vi "Thermometer_Property Node Demo.vi"() -> ()   [LabVIEW 2010]
panel:
  in  "Stop Button":bool
  in  "Temperature":dbl format="%.2g"
  out "Thermometer":dbl(slide) scale=0.0..100.0
  # "The color of the thermometer changes\nwhen the temperature is above 50 degrees."
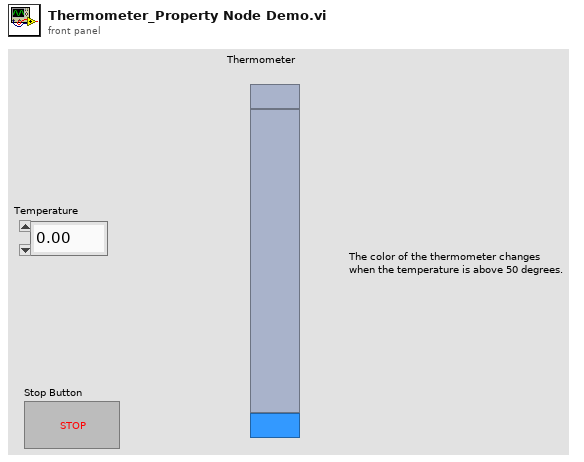
[diagram p1: front panel]
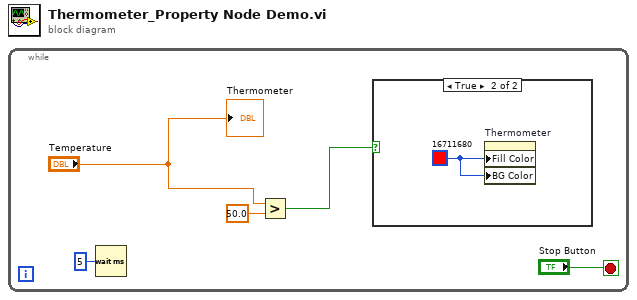
[diagram p0: block diagram]
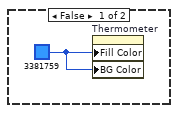
[diagram p2: hidden frame]
diagram:
  n1 = while {
    stop <- "Stop Button" stop-if-true
    n2 = Wait (ms)(milliseconds to wait=u32 5) -> ()  [unwired: 1 out]
    n3 = Greater?(x="Temperature", y=50.0) -> (0:w2:bool)
    n4 = case shown="True" w2 {
      frame False {
        w6 = u32 3381759
        n5 = property on="Thermometer" class="Slide (strict)"("Fill Color"=w6, "BG Color"=w6) -> ()  [unwired: 2 in, 2 out]
      }
      frame True {
        w7 = u32 16711680
        n6 = property on="Thermometer" class="Slide (strict)"("Fill Color"=w7, "BG Color"=w7) -> ()  [unwired: 2 in, 2 out]
      }
    }
    "Thermometer" <- "Temperature"
  }
